vi "Result-Evaluate.vi"() -> ()   [LabVIEW 2020]
doc: "This example demonstrates how to continuously acquire thermocouple measurements using a DAQmx device.\n\nFor instructions on how to connect your signals to the DAQ device, refer to your device documentation."
uses:
  RandI8.vi
  <vilib>/GPower/Numeric/GPNumeric.lvlib
panel:
  out "Max":dbl format="%#.2f"
  out "Mean":dbl format="%#.2f"
  out "Variance":dbl format="%#.2f"
  out "Standard Deviation":dbl format="%#.2f"
  out "Min":dbl format="%#.2f"
  out "XY Graph":cluster{i32[], i8[]}(graph)
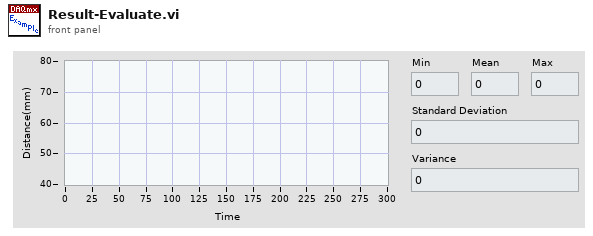
[diagram p1: front panel]
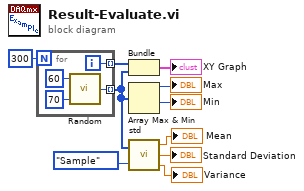
[diagram p0: block diagram]
diagram:
  n1 = for {
    N: 300 -> [_]
    tunnel: [w12] -> w3 mode=indexing
    tunnel: [w11] -> w8 mode=indexing
    i -> [w11]
    n2 = call-poly <vilib>:"Random.vi"("Limit b"=i8 70, "Limit a"=i8 60) -> ("Random number"=w12:i8)  [unwired: 3 in]
  }
  n3 = Bundle(w8, w3) -> (→"XY Graph":cluster{i32[], i8[]})  [unwired: 1 in]
  n4 = Array Max & Min(array=w3) -> (max value=→"Max":i8, min value=→"Min":i8)  [unwired: 2 out]
  n5 = call "std.vi"("X"=w3, "Weighting (Sample)"=enum16{"Sample", "Population"}."Sample") -> ("mean"=→"Mean":dbl, "Standard Deviation"=→"Standard Deviation":dbl, "Variance"=→"Variance":dbl)
